vi "UHR-Fleezers Control (host) - Lorentz v4.vi"() -> ()   [LabVIEW 2014] (continued)
  out "Amp current":dbl[](graph)=[0.0169526657918025, 0.016960112308114644, 0.0169526657918025, 0.016960112308114644, 0.016932645649586246, 0.01696502578814028, 0.016922727134006547, 0.01697497482222945, 0.016955534531693243, 0.016920682393871657, 0.016913052766502658, 0.016956877346110188, 0.01690490432447257, 0.016908047730948596, 0.016886989959410157, 0.0168990142521437, 0.016891079439679938, 0.016886379589220638, 0.016868465224158226, 0.016933408612323148, 0.01688827173680815, 0.01690227973265763, 0.016862422559281977, 0.016931455427716683, 0.01689678640095195, 0.016911008026367767, 0.016896206549271906, 0.01695397808770997, 0.016912045655689947, 0.016928769798882796, 0.0169044770653399, 0.01693642994476127, 0.016903012176885054, 0.01690923795281816, 0.016908627582628635, 0.016958189642017656, 0.0169203772087769, 0.016929624317148124, 0.01689678640095195, 0.016945371868037736, 0.01693932920316149, 0.016923978392895066, 0.016900112918484835, 0.016959105197301934, 0.01693551438947699, 0.016914761803033314, 0.016874019592882858, 0.016916684469130302, 0.016878353221228447, 0.016893490401928547, 0.01686446729941687, 0.01691998046815371, 0.016895077364421293, 0.016919797357096856, 0.016901242103335445, 0.016928983428449125, 0.016912137211218377, 0.016924344615008777, 0.016907071138645362, 0.016948728904080095, 0.01691830195013253, 0.016923215430158164, 0.01688412121951941, 0.016954222235785774, 0.016917874690999864, 0.016929868465223933, 0.017037171544541534, 0.017055513168736606, 0.01704351939451254, 0.01703344828638546, 0.017046937467573853, 0.017029999694814675, 0.017005127109591737, 0.017014557329019818, 0.017042481765190357, 0.01701828058717589, 0.01702325510422048, 0.01703155613879795, 0.017028443250831398, 0.017003631702627413, 0.017003540147098987, 0.017018677327799075, 0.017034058656574983, 0.017009674367503662, 0.017002533036286276, 0.017015076143680908, 0.017031495101779, 0.017036103396709874, 0.017019562364573883, 0.01703680532242782, 0.01703247169408223, 0.017042023987548217, 0.017036347544785682, 0.017039704580828038, 0.017048371837519224, 0.017023987548447903, 0.017018555253761176, 0.01701858577227065, 0.05867714468825214, 0.05870891445661666, 0.058683095797599956, 0.05870555742057429, 0.058757133701588735, 0.058661000396739334, 0.05859691152683975, 0.05860075685903373, 0.058646565141757194, 0.05849485763115201, 0.05836561174352117, 0.05846021912289676, 0.05851405377361242, 0.058334055604723, 0.05814590899380348, 0.05832355723746325, 0.05841291543320897, 0.058184301278724274, 0.0581402935880599, 0.05840501113925468, 0.058464674825280255, 0.05835297708059811, 0.05824994659260716, 0.058513657032989226, 0.058697958311714774, 0.05858626056703263, 0.058617084261603385, 0.05881652272102902, 0.058878688924831626, 0.0588497268593389, 0.05885311441389074, 0.05887240211187957, 0.058940702536086846, 0.05897109897152494, 0.05889873958555736, 0.05887862788781267, 0.0589223303933823, 0.058909298989836045, 0.058916440321053434, 0.05885915707876699, 0.058968779564804764, 0.05885961485640912, 0.05876015503402685, 0.05881301309243928, 0.05886797692800556, 0.05875923947874257, 0.05869737846003473, 0.05872920926541819, 0.058807306131167275, 0.058688192388682454, 0.05864888454847737, 0.058773033845025725, 0.05883294167912711, 0.05877095858638136, 0.05871828363902579, 0.05878093813898001, 0.0589785149693276, 0.058929837946713394, 0.05889736625263094, 0.058995330668048886, 0.059074068422496955, 0.05902313303018152, 0.05905365153965752, 0.05902941984313356, 0.05876702169865896, 0.05880504776146604, 0.058806085390788236, 0.05879586169011377, 0.05884539323099332, 0.0588626972258662, 0.05887383648182495, 0.05881914731284396, 0.058912625507368935, 0.05881188390758866, 0.05869289223914176, 0.05873934141056422, 0.05880053102206359, 0.058644154179508586, 0.05851768547624006, 0.058613818781089455, 0.058685048982206424, 0.058522659993284654, 0.05842268135624129, 0.05860997344889547, 0.05869811090426215, 0.058628986480299024, 0.05857280190435372, 0.05869985045930229, 0.058889126255072415, 0.05879457991271578, 0.058788689840386904, 0.05892318491164763, 0.058971831415752365, 0.05892013306070003, 0.05893545335245698, 0.058890041810356696, 0.05878170110171691, 0.058839197973569686, 0.05883425397503458, 0.05883999145481606, 0.058881496627703415, 0.058851222266303224, 0.058815057832574166, 0.058749748222295534, 0.05883022553178374, 0.05875231177709152, 0.058630390331734915, 0.05871446882534128, 0.0587492904446534, 0.05856462294381415, 0.05845246742148986, 0.05858781701101591, 0.058693929868463945, 0.05851161229285434, 0.05842631305886894, 0.058632129886775054, 0.05872634052552745, 0.05861891537217195, 0.058535142063660325, 0.058678090762045894, 0.058843440046386856, 0.05878841517380163, 0.05875688955351293, 0.058908078249457006, 0.05898879970702102, 0.058959288308357734, 0.058988036744284114, 0.05898190252387944, 0.058596240119631285, 0.058748527481916495, 0.05874556718649733, 0.058761345255896415, 0.05880101931821521, 0.0588375194555485, 0.058903530991545085, 0.0587775200659187, 0.058887234107484906, 0.058839869380778155, 0.058704184087647875, 0.058698568681904296, 0.058713827936642295, 0.0585772576067372, 0.05845738090151549, 0.05850675984984766, 0.05861015655995234, 0.058485671559799744, 0.05842185735648543, 0.058601214636675864, 0.058648121585740474, 0.05859996337778734, 0.05855214087343846, 0.058672566911830745, 0.05884759056367559, 0.05878975798821857, 0.05877803888057979, 0.05885317545090969, 0.058908474990080194, 0.05888726462599438, 0.05890273751029871, 0.058803399761954346, 0.05871681875057094, 0.05878859828485848, 0.058835230567337804, 0.05886474196600109, 0.0589122898037647, 0.05887401959288179, 0.058873134556106994, 0.05876183355204803, 0.05887066255683944, 0.05875139622180725, 0.0586343577379668, 0.05867735831781847, 0.05873665578173034, 0.0585823541978197, 0.058473769341104105, 0.0585251319925522, 0.058599078341012543, 0.05843836787011195, 0.058349772637103135, 0.05851222266304386, 0.058603686635943425, 0.05852912991729356, 0.05853346354563915, 0.0586587725455476, 0.05880602435376927, 0.05876897488326542, 0.05873751029999567, 0.05881136509292758, 0.05890054017761644, 0.058819757683033484, 0.05879860835596661, 0.05880217902157531, 0.05889974669637006, 0.05896551408429084, 0.058984923856317574, 0.05896411023285493, 0.05903811761833423, 0.059025818659015405, 0.05908288827173551, 0.05897918637653608, 0.059064699240087816, 0.05897958311715927, 0.05885155796990746, 0.05884398937955741, 0.05889040803247041, 0.05873070467238251, 0.05861577196569592, 0.058758232367929875, 0.05888384655293307, 0.05866118350779621, 0.05851628162480418, 0.05870332956938255, 0.05880050050355412, 0.058731589709157324, 0.05870787682729447, 0.058827570421459335, 0.058956511123995414, 0.058872737815483814, 0.058847376934109255, 0.058931089205601916, 0.05896514786217713, 0.058957976012450265, 0.05900302133243683, 0.05900717184972557, 0.06101351969969651, 0.06100839259010454, 0.0610315866573063, 0.06104242072817028, 0.061070741904964004, 0.061021759697255026, 0.06087478255561864, 0.06096603289895187, 0.061050904873804594, 0.06088381603442353, 0.060784295175022304, 0.06089385662404114, 0.06096615497298976, 0.0607882320627447, 0.0605131076998186, 0.06074556718649726, 0.06088857692190178, 0.06070140690328549, 0.0607113254188652, 0.060980132450329766, 0.06108334604937759, 0.06106183050019703, 0.0610269173253565, 0.06115659047211998, 0.06127973265785563, 0.061202185125277114, 0.06119818720053577, 0.06126438184758922, 0.06133845027008745, 0.0613045747245691, 0.06130579546494813, 0.06127933591723245, 0.05855381939145965, 0.05864778588213623, 0.05864717551194672, 0.05865880306405707, 0.05868761253700241, 0.058670949430828526, 0.05869023712881735, 0.05858568071535258, 0.05865987121188873, 0.058558824427013705, 0.05844840845972956, 0.05845713675343968, 0.05853523361918876, 0.0584093142490908, 0.05830329294717119, 0.05836045411541973, 0.05842518387401832, 0.05830616168706193, 0.058225074007384206, 0.05840299691762928, 0.05847492904446419, 0.058402478102968176, 0.058411206396678315, 0.05852949613940728, 0.058743308816796104, 0.058691610461743766, 0.05866734824671034, 0.05872603534043269, 0.05876793725394323, 0.05870751060518076, 0.05876030762657424, 0.05872774437696335, 0.058540604876856535, 0.05860780663472268, 0.05859538560136596, 0.05858815271462014, 0.05863768425549967, 0.0585609912411865, 0.05847074800866599, 0.058447645496992655, 0.05850093081453774, 0.05836039307840078, 0.05823578600421028, 0.058302194280830055, 0.05836890774254458, 0.05820865504928613, 0.05803341776787497, 0.05822223578600294, 0.058326456495863474, 0.05810513626514355, 0.05803088473158845, 0.058302224799339525, 0.05838605914487009, 0.05830237739188691, 0.05823041474654251, 0.05844843897823903, 0.058613361003447315, 0.05853691213720995, 0.05851008636738054, 0.05862434766685867, 0.05869426557206819, 0.05865959654530345, 0.058693014313179664, 0.05867390972624769, 0.058459608752707254, 0.058497940000609094, 0.058514297921688226, 0.05845851008636611, 0.058465498825036114, 0.05839936521500163, 0.05831144138920129, 0.05836378063295261, 0.058509659108247875, 0.05833979308450448, 0.05816058839686143, 0.05820911282692826, 0.058273018585771004, 0.058127506332589465, 0.05791500595110811, 0.058098239082001964, 0.05819550157170197, 0.05795974608599991, 0.05790282906582718, 0.05815613269447793, 0.05821353801080229, 0.05813074129459392, 0.05802249214148255, 0.0582559892574834, 0.05843949705496257, 0.058309305093537954, 0.05832450331125701, 0.0584761803033527, 0.058528916287727224, 0.058529068880274614, 0.05852293465986993, 0.058511825922420664, 0.05836075930051449, 0.05838044373912651, 0.05834656819360815, 0.0583083590197442, 0.05836790063173187, 0.0583271889400909, 0.05821387371440652, 0.05820007934812337, 0.05828766747031948, 0.05810458693197297, 0.05798095645008572, 0.058052858058411164, 0.058106570635088915, 0.057952635273292, 0.05776818140201908, 0.05797247230445139, 0.058080294198430076, 0.057839930417797156, 0.057788201544235335, 0.058037812433239494, 0.058113742484815774, 0.05804470961638108, 0.05790942106387399, 0.05814114810632523, 0.05830320139164276, 0.05820310068056149, 0.05820941801202303, 0.05836936552018671, 0.05845033112582654, 0.0584423657948533, 0.05845237586596143, 0.05843824579607405, 0.06618018127994545, 0.06624231696523857, 0.06621686452833558, 0.066234138004699, 0.06623569444868228, 0.0661422162541573, 0.06606472975859774, 0.0660725424970236, 0.06616202276680722, 0.06602536088137372, 0.06589510788293017, 0.06595434430982307, 0.0660394909512611, 0.06588830225531703, 0.06573943296609311, 0.0658894619586771, 0.06600634784997017, 0.06578795739615995, 0.0657112338633373, 0.06595065157017647, 0.06601303140354542, 0.0659321878719435, 0.06585607470931037, 0.06604416028321092, 0.06619989623706693, 0.06608703878902471, 0.06609637745292435, 0.06622721030304794, 0.06632587664418385, 0.06631598864711362, 0.06632871486556512, 0.06636286507766875, 0.05736872463148777, 0.0574271675771343, 0.05746177556688008, 0.05744721823786003, 0.057509079256567876, 0.05756801049836602, 0.05761238441114413, 0.057530045472577875, 0.05764592425305824, 0.057585131382182055, 0.05749800103762809, 0.05745878475295143, 0.05749580370494582, 0.0574180120242915, 0.05724723044526382, 0.057307199316384165, 0.05737723929563157, 0.05723194067201635, 0.05720749534592608, 0.05727069917905087, 0.057326944792015125, 0.05728937650685018, 0.05714386425366863, 0.05728485976744773, 0.05739963988158695, 0.05727668080690817, 0.057335856196782116, 0.057406933805351716, 0.05750538651692127, 0.05751487777336831, 0.05750791955320778, 0.05751237525559128, 0.0579019135105429, 0.057950621051666575, 0.05796240119632431, 0.05800354014709795, 0.05807751701406777, 0.05802401806695634, 0.05797326578569777, 0.05794228949857964, 0.05806445509201205, 0.057933103427227364, 0.05782091738639359, 0.05785024567400003, 0.05789986877040799, 0.05782879116183841, 0.05771279030732014, 0.057787591174045805, 0.05788631855220066, 0.05776650288399789, 0.05774541459394999, 0.05785424359874138, 0.05789892269661424, 0.057857509079255326, 0.05777422406689533, 0.05784292123172579, 0.05801474044007564, 0.057907681508833846, 0.05787569811090301, 0.057927182836389014, 0.05803646961882255, 0.05800271614734211, 0.05796234015930536, 0.0580202642902908, 0.05792464980010252, 0.05796942045350379, 0.05797836237678025, 0.05799984740745135, 0.0580758384960466, 0.058039918210393344, 0.05797555467390846, 0.057967711416973135, 0.05806714072084593, 0.05790752891628647, 0.05781246375926873, 0.05789739677114044, 0.05790667439802114, 0.05778249458296332, 0.05767168187505598, 0.05778655354472362, 0.05789397869807913, 0.0577122104556401, 0.05768956572160892, 0.05784655293435343, 0.05788677632984279, 0.05784020508438243, 0.05778206732383066, 0.057885952330086934, 0.05803570665608565, 0.05795416119876579, 0.057946226386302035, 0.05803753776665421, 0.05812762840662736, 0.058096713156528174, 0.05809207434308782, 0.058102298043762275, 0.05806143375957393, 0.05811123996703875, 0.05805520798364082, 0.058111789300209306, 0.05817474898525829, 0.0580753196813855, 0.058212408825951675, 0.058142857142855886, 0.058066560869165895, 0.05824359874263614, 0.05785604419080046, 0.05796322519608016, 0.05793871883297095, 0.05772667622913172, 0.05788586077455851, 0.05762819299905268, 0.05773351237525435, 0.05785674611651842, 0.057791344950711344, 0.05774202703939816, 0.057862514114809395, 0.05796548356578139, 0.058087252418590606, 0.05802334665974788, 0.058187139500105546, 0.05831589709158477, 0.058206366161075426, 0.05834241767631942, 0.058355296487318284, 0.05832770775475199, 0.058404431287574644, 0.05832322153385901, 0.057956236457410173, 0.05807815790276677, 0.05797738578447702, 0.05809973448896629, 0.058119327372049896, 0.05800067140720722, 0.058170628986479025, 0.05800714133121612, 0.058036286507765704, 0.05824527726065733, 0.057814294869837295, 0.05800772118289617, 0.057920133060700076, 0.057680990020446146, 0.0579498275704202, 0.05751332132938503, 0.05765117343668811, 0.05784679708242925, 0.05769692068239263, 0.057814172795799416, 0.05789358195745595, 0.05794454786828085, 0.05816174810022152, 0.058005859553818144, 0.05820203253272983, 0.05834952848902733, 0.05815979491561506, 0.058378124332406335, 0.05834629352702286, 0.058285500656146676, 0.058417096469007175, 0.05825724051637192, 0.00451747184667494, 0.0045178380687886524, 0.004530625324259094, 0.004513870662556772, 0.004487319559312655, 0.00448576311532938, 0.004487960448011651, 0.004507248146000482, 0.004523758659626995, 0.004526871547593547, 0.004501358073671614, 0.00451976073488564, 0.004508896145512186, 0.004513260292367252, 0.004468642231513346, 0.004494369335001612, 0.0045054170354319216, 0.004491683706167724, 0.004517441328165464, 0.004521317178868915, 0.0044969328897975945, 0.00449894711142301, 0.004529099398785295, 0.004523361919003807, 0.0044921414838098635, 0.004499893185216767, 0.004504501480147641, 0.004517807550279176, 0.004495254371776414, 0.0045184179204686955, 0.004501815851313753, 0.004515915402691664, 0.00451518295846424, 0.004509201330606945, 0.004514664143803148, 0.0045286111026336786, 0.0045125583666493045, 0.004529648731955862, 0.0045194860683003555, 0.004531632435071802, 0.004528153324991538, 0.0045108493301186485, 0.004501663258766373, 0.004521774956511055, 0.004506179998168821, 0.004507034516434149, 0.00453736991485329, 0.004532212286751846, 0.004493789483321567, 0.004512192144535593, 0.004510544145023889, 0.0045054170354319216, 0.004482680745872304, 0.004494644001586895, 0.004525864436780839, 0.004527573473311494, 0.004488357188634839, 0.004510727256080744, 0.004482375560777544, 0.004494460890530039, 0.004530747398296998, 0.004528153324991538, 0.0045117038483839765, 0.004530106509598003, 0.004536667989135342, 0.004536973174230101, 0.004502456740012749, 0.004504898220770829, 0.0045134128849146325, 0.004523422956022759, 0.004539872432630321, 0.004540787987914601, 0.004515091402935813, 0.0045239112521743745, 0.0045441755424664365, 0.00454490798669386, 0.004507156590472053, 0.0045294045838800544, 0.00454506057924124, 0.0045275429548020186, 0.004537614062929097, 0.004557512131107447, 0.00454261909848316, 0.004543076876125301, 0.004543870357371677, 0.004556077761162075, 0.004526810510574595, 0.0045342570268867375, 0.004537766655476477, 0.004520157475508827, 0.004520004882961447, 0.004536881618701674, 0.004530930509353854, 0.0045216223639636755, 0.004538926358836565, 0.004546220282601328, 0.00453050325022119, 0.004536637470625865, 0.004538438062684949, 0.004536362804040581, 0.004521897030548959, 0.00454261909848316, 0.004539201025421849, 0.004540604876857745, 0.004533066805017174, 0.0045422528763694485, 0.0045353251747183975, 0.004539353617969229, 0.004543412579729536, 0.00453172399060023, 0.004509842219305941, 0.004526566362498786, 0.004526139103366122, 0.004507553331095241, 0.004505935850093013, 0.004508407849360569, 0.004485183263649335, 0.004518478957487648, 0.004524857325968131, 0.004523148289437475, 0.0044967192602312625, 0.004523636585589091, 0.004524063844721755, 0.004527634510330446, 0.004510238959929129, 0.4378774681844542, 1.1794734031189942, 1.1789416180913743, 1.1792670369579177, 1.179584032715845, 1.1793981749931346, 1.1797783135471682, 1.1800726035340454, 1.1801462141789023, 1.1801267433698555, 1.1802436597796602, 1.1802706991790544, 1.1801345561082817, 1.1798594622638647, 1.1805548570207856, 1.1800792870876216, 1.180210882900482, 1.1803491927854268, 1.180768028809476, 1.1809785149693315, 1.180827448347424, 1.1799802240058617, 1.179896664326917, 1.180044587542347, 1.1803296304208517, 1.1806996978667577, 1.1806953337199022, 1.1803043610950055, 1.1801087679677742, 0.004506088442640393, 0.0045059968871119654, 0.004491286965544535, 0.004513748588518868, 0.004526596881008263, 0.004524460585344943, 0.004505478072450874, 0.004522293771172147, 0.004515152439954764, 0.004519241920224548, 0.004482039857173309, 0.0044971465193639265, 0.004498001037629254, 0.0045084994048889965, 0.004515121921445288, 0.004521164586321535, 0.004507797479171049, 0.004512009033478736, 0.004528153324991538, 0.00452836695455787, 0.004506271553697249, 0.004514511551255768, 0.004501449629200041, 0.004526291695913503, 0.004532151249732895, 0.0045214087343973435, 0.004510788293099696, 0.004531937620166562, 0.004528855250709486, 0.004528794213690534, 0.004525589770195555, 0.0045243385113070385, 0.0045346842860194015, 0.004532090212713943, 0.004516800439466468, 0.004500595110934714, 0.004492385631885671, 0.004502883999145414, 0.004513321329386205, 0.004511154515213408, 0.004502151554917989, 0.00450840784936057, 0.004521225623340487, 0.004522293771172147, 0.004514236884670484, 0.004512466811120877, 0.004515396588030573, 0.004535660878322634, 0.004548966948454168, 0.004552293465987052, 0.004536149174474249, 0.004540818506424077, 0.00451960814233826, 0.004544022949919057, 0.004505386516922445, 0.004527726065858875, 0.004533524582659314, 0.0045262611774040265, 0.004496505630664931, 0.00451686147648542, 0.004499343852046198, 0.00450672933133939, 0.004491500595110867, 0.004498580889309298, 0.004497970519119779, 0.004507980590227906, 0.004519058809167692, 0.00452714621417883, 0.004487655262916892, 0.004493240150150999, 0.004516464735862233, 0.0045340433973204055, 0.004503250221259125, 0.004529648731955862, 0.00453141880550547, 0.004522385326700575, 0.004505172887356113, 0.0045101474044007, 0.004472151860103085, 0.004482497634815448, 0.004503311258278077, 0.004508224738303713, 0.004481734672078548, 0.004476821192052912, 0.00448133793145536, 0.0044705343791008574, 0.004461653492843343, 0.004484511856440865, 0.0044708090456861424, 0.004477065340128721, 0.004498916592913535, 0.0045179906613360315, 0.004504165776543405, 0.004503036591692794, 0.004511093478194457, 0.004509109775078518, 0.004491317484054011, 0.0044997100741599105, 0.004502395702993798, 0.004528489028595774, 0.004513290810876728, 0.004509414960173277, 0.004487166966765276, 0.004490585039826587, 0.004505539109469825, 0.004507461775566813, 0.004499343852046199, 0.00451350444044306, 0.004525437177648175, 0.004515549180577952, 0.004484939115573528, 0.004506698812829914, 0.004477126377147673, 0.004498092593157682, 0.0045196996978666875, 0.004511307107760788, 0.004494491409039515, 0.004516220587786424, 0.00448377941221344, 0.0044651020844141305, 0.004472701193273654, 0.004486190374462044, 0.004484633930478769, 0.0044800866725668445, 0.004447065645313817, 0.004473952452162169, 0.004472640156254701, 0.004481032746360601, 0.004478347117526713, 0.004480666524246888, 0.004484664448988244, 0.004488845484786455, 0.004467726676229066, 0.004478499710074093, 0.004464552751243563, 0.004477187414166625, 0.004497085482344975, 0.0044811548203985046, 0.0044492629779960885, 0.00446327097384557, 0.0044792321543015165, 0.004483260597552348, 0.004469466231269198, 0.004472518082216797, 0.004504104739524454, 0.00449125644703506, 0.00450169377727585, 0.004497054963835498, 0.00446632282479317, 0.00447212134159361, 0.004497482222968162, 0.004509384441663801, 0.004476973784600293, 0.004497634815515542] caption="Most Recent Time Trace"
  out "Values":dbl[](array[numeric])=[nan, nan, 0.010932615131076998, nan, nan, 0.010855525376140629, -inf, 0.0332469252601703, -inf, 0.03308018738364819, nan, nan, 0.005625431073946348, 0.01681456484606091, 0.0867058284381119, 1.1533333333333333]
  out "All Signals":waveform(dbl)[](graph)=[{"t0"=timestamp(317.7000000000063 s since 1904-01-01), "dt"=0.15, "Y"=[0.0, 0.0], "attributes"=variant("NI_ChannelName"=variant(string "APD 1"))}, {"t0"=timestamp(317.7000000000063 s since 1904-01-01), "dt"=0.15, "Y"=[0.0, 0.0], "attributes"=variant("NI_ChannelName"=variant(string "APD 2"))}, {"t0"=timestamp(317.7000000000063 s since 1904-01-01), "dt"=0.15, "Y"=[0.0, 0.0], "attributes"=variant("NI_ChannelName"=variant(string "APD 3"))}, {"t0"=timestamp(317.7000000000063 s since 1904-01-01), "dt"=0.15, "Y"=[nan, nan], "attributes"=variant("NI_ChannelName"=variant(string "T1 Y"))}, {"t0"=timestamp(317.7000000000063 s since 1904-01-01), "dt"=0.15, "Y"=[nan, nan], "attributes"=variant("NI_ChannelName"=variant(string "T1 X"))}, {"t0"=timestamp(317.7000000000063 s since 1904-01-01), "dt"=0.15, "Y"=[0.010935636463514926, 0.01092959379863868], "attributes"=variant("NI_ChannelName"=variant(string "T1 Sum"))}, {"t0"=timestamp(317.7000000000063 s since 1904-01-01), "dt"=0.15, "Y"=[nan, nan], "attributes"=variant("NI_ChannelName"=variant(string "T2 Y"))}, {"t0"=timestamp(317.7000000000063 s since 1904-01-01), "dt"=0.15, "Y"=[nan, nan], "attributes"=variant("NI_ChannelName"=variant(string "T2 X"))}, {"t0"=timestamp(317.7000000000063 s since 1904-01-01), "dt"=0.15, "Y"=[0.010837214270454837, 0.010873836481826035], "attributes"=variant("NI_ChannelName"=variant(string "T2 Sum"))}, {"t0"=timestamp(317.7000000000063 s since 1904-01-01), "dt"=0.15, "Y"=[-inf, -inf], "attributes"=variant("NI_ChannelName"=variant(string "T1 FB X"))}, {"t0"=timestamp(317.7000000000063 s since 1904-01-01), "dt"=0.15, "Y"=[0.03323676259651433, 0.033257087923825326], "attributes"=variant("NI_ChannelName"=variant(string "T1 FB Sum"))}, {"t0"=timestamp(317.7000000000063 s since 1904-01-01), "dt"=0.15, "Y"=[-inf, -inf], "attributes"=variant("NI_ChannelName"=variant(string "T2 FB X"))}, {"t0"=timestamp(317.7000000000063 s since 1904-01-01), "dt"=0.15, "Y"=[0.033094546342356174, 0.03306582842493926], "attributes"=variant("NI_ChannelName"=variant(string "T2 FB Sum"))}, {"t0"=timestamp(317.7000000000063 s since 1904-01-01), "dt"=0.15, "Y"=[nan, nan], "attributes"=variant("NI_ChannelName"=variant(string "T3 Y"))}, {"t0"=timestamp(317.7000000000063 s since 1904-01-01), "dt"=0.15, "Y"=[nan, nan], "attributes"=variant("NI_ChannelName"=variant(string "T3 X"))}, {"t0"=timestamp(317.7000000000063 s since 1904-01-01), "dt"=0.15, "Y"=[0.005610065004425081, 0.005640797143467409], "attributes"=variant("NI_ChannelName"=variant(string "T3 Sum"))}, {"t0"=timestamp(317.7000000000063 s since 1904-01-01), "dt"=0.02, "Y"=[0.015748031496062992, 0.015748031496062992, 0.015748031496062992, 0.015748031496062992, 0.015748031496062992, 0.015748031496062992, 0.015748031496062992, 0.015748031496062992, 0.015873015873015872, 0.023622047244094488, 0.015873015873015872, 0.015748031496062992, 0.023622047244094488, 0.015748031496062992, 0.015748031496062992], "attributes"=variant("NI_ChannelName"=variant(string "PSD X"))}, {"t0"=timestamp(317.7000000000063 s since 1904-01-01), "dt"=0.02, "Y"=[0.08661417322834646, 0.08661417322834646, 0.08661417322834646, 0.08661417322834646, 0.08661417322834646, 0.08661417322834646, 0.08661417322834646, 0.08661417322834646, 0.0873015873015873, 0.08661417322834646, 0.0873015873015873, 0.08661417322834646, 0.08661417322834646, 0.08661417322834646, 0.08661417322834646], "attributes"=variant("NI_ChannelName"=variant(string "PSD Y"))}, {"t0"=timestamp(317.7000000000063 s since 1904-01-01), "dt"=0.02, "Y"=[1.1545454545454545, 1.1545454545454545, 1.1545454545454545, 1.1545454545454545, 1.1545454545454545, 1.1545454545454545, 1.1545454545454545, 1.1545454545454545, 1.1454545454545455, 1.1545454545454545, 1.1454545454545455, 1.1545454545454545, 1.1545454545454545, 1.1545454545454545, 1.1545454545454545], "attributes"=variant("NI_ChannelName"=variant(string "PSD Sum"))}]
  in  "PSD downsample":dbl=1.0 caption="PSD Downsample" min=1.0 max=5.0
  in  "Signals to Plot":i32(listbox)=18
  out "Trap Disp. Freq. (Hz)":dbl=6.666666666666667 caption="Freq. (Hz)" format="%#_6p"
  out "Display Period (s)":dbl=0.15 caption="Period (s)" format="%#_6p"
  in  "Trap Disp. Downsample":dbl=10000.0 caption="Downsample" max=20000.0
  in  "APD Disp. Scale":dbl=0.1 caption="Scale (Divide,\nfor above plot only)"
  in  "APD Disp. Downsample":dbl=150.0 caption="Integrate" max=300.0
  out "APD Display Freq. (Hz)":dbl=6.666666666666667 caption="Freq. (Hz)"
  out "APD Display Period (s)":dbl=0.15 caption="Period (s)"
  out "FFT 1":cluster{"f0":dbl, "df":dbl, "magnitude":dbl[]}[](graph)=[{"f0"=0.0, "df"=3.3333333333333335, "magnitude"=array[10000 elements]}, {"f0"=0.0, "df"=3.3333333333333335, "magnitude"=array[10000 elements]}]
  out "FFT 2":cluster{"f0":dbl, "df":dbl, "magnitude":dbl[]}[](graph)
  in  "FFT 1 Choice 1":u16(ring) items=["T1 Y", "T1 X", "T1 Sum", "T2 Y", "T2 X", "T2 Sum", "T1 FB X", "T1 FB Sum", "T2 FB X", "T2 FB Sum", "PSD Y", "PSD X", "PSD Y Sum", "none"]
  in  "FFT 2 Choice 1":u16(ring)=13 items=["T1 Y", "T1 X", "T1 Sum", "T2 Y", "T2 X", "T2 Sum", "T1 FB X", "T1 FB Sum", "T2 FB X", "T2 FB Sum", "PSD Y", "PSD X", "PSD Y Sum", "none"]
  in  "FFT 1 Choice 2":u16(ring)=1 items=["T1 Y", "T1 X", "T1 Sum", "T2 Y", "T2 X", "T2 Sum", "T1 FB X", "T1 FB Sum", "T2 FB X", "T2 FB Sum", "PSD Y", "PSD X", "PSD Y Sum", "none"]
  in  "FFT 2 Choice 2":u16(ring)=13 items=["T1 Y", "T1 X", "T1 Sum", "T2 Y", "T2 X", "T2 Sum", "T1 FB X", "T1 FB Sum", "T2 FB X", "T2 FB Sum", "PSD Y", "PSD X", "PSD Y Sum", "none"]
  in  "Compute FFT":bool
  in  "Reset FFT":bool
  in  "# Spectra to Ave.":dbl=25.0
  out "Ave. Time (s)":dbl=7.5
  out "1 Channel":waveform(dbl)(graph)={"t0"=timestamp(0 s since 1904-01-01), "dt"=1.4999999999999999e-05, "Y"=array[20000 elements], "attributes"=variant("NI_ChannelName"=variant(string "T1 X"))}
  out "Slow mean":dbl=nan format="%0.2f"
  in  "Slow mean N ave.":dbl=1.0 min=1.0 step=1.0
  out "Mean Intensity":dbl=nan
  out "Sigma":dbl=nan
  out "Sigma/Mean":dbl=nan
  in  "Subtract mean":bool
  in  "High Res. Display":u16(ring)=1 items=["T1 Y", "T1 X", "T1 Sum", "T2 Y", "T2 X", "T2 Sum", "T1 FB X", "T1 FB Sum", "T2 FB X", "T2 FB Sum", "PSD Y", "PSD X", "PSD Y Sum"]
  in  "Tab Control":T7(tab)=enum."Trap Control (RF)"
  in  "Visa resource for valves":refnum<visa-resource-name>="COM10"
  in  "Cursor control":cluster{"X":bool, "Y":bool}
  in  "Trap 3 (ON/OFF)":bool=TRUE
  in  "Maximum Delta\n(MHz)":dbl=30.0
  in  "T3 Y (V)":dbl min=0.0 max=10.0 step=1.0 format="%#_6f"
  in  "T3 X (V)":dbl=3.0 min=0.0 max=10.0 step=1.0 format="%#_6f"
  in  "Shunt 1":bool caption="Inject Pump 3"
  in  "manual raster set":u16(ring) items=["offset", "user-defined", "basepaire step", "user-defined 2", "user-defined 3", "user-defined 4"]
  in  "move Con X?":bool
  in  "Symmetric?":bool
  out "Laser Intensity Low (bugs to fix)":bool
  out "Good freq?":bool=TRUE
  in  "T2 calibration":T8 {"T2 kappa_x (pN/nm)" min=0.0 step=0.001 format="%#_2g"; "T2 offset_x (mV)" format="%#_2g"; "T2 alpha_x (nm/V)" step=10.0 format="%#_3g"}
  in  "T1 calibration":T9 {"T1 kappa_x (pN/nm)" min=0.0 step=0.001 format="%#_2g"; "T1 offset_x (mV)" format="%#_2g"; "T1 alpha_x (nm/V)" step=10.0 format="%#_3g"}
  in  "Blue FB Setpoint (mV)":dbl=90.0
  in  "Blue Laser ON":bool
  in  "11":bool
  out "Stage Moving":bool
  in  "Read Cal":bool
  in  "Speed (nm/s)":dbl=100.0
  in  "Furthest Withdraw (MHz)":dbl=15.0
  in  "Round T1 X":bool caption="Round"
  in  "Cal sets to save":u32=25 min=1 step=1
  in  "Trap 2 (ON/OFF)":bool=TRUE
  in  "Trap 1 (ON/OFF)":bool=TRUE
  in  "Save Calibration":bool
  out "Manipulating Trap":bool
  out "Buffer Status":dbl(slide) scale=0.0..1.0
  out "Overflow (data lost)":bool
  in  "Reset":bool
  out "Data Rate (Hz)":dbl=66666.66666666667 caption="Trap Data Rate (Hz)" format="%#_3p"
  out "Data Period (s)":dbl=1.4999999999999999e-05 caption="Trap Data Period (s)" format="%#_6p"
  in  "BD 1 Frequency 1 (MHz)":dbl=75.0 caption="T1 X (MHz)" min=60.0 max=90.0 step=1.0 format="%#_6p"
  in  "BD 1 Frequency 2 (MHz)":dbl=90.0 caption="T2 X (MHz)" min=60.0 max=90.0 step=1.0 format="%#_6p"
  in  "Round T2 X":bool caption="Round"
  in  "Trap Raster Scan":bool
  out "Raster Scanning...":bool
  in  "Trap Delta (MHz)":dbl=15.0
  in  "Setpoints (V)":cluster{"Set 1":dbl, "Set 2":dbl}={"Set 1"=0.9, "Set 2"=0.9}
  in  "Fish for Tether":bool
  in  "Red FB Setpoint (mV)":dbl=100.0
  in  "Confocal Linescan":bool
  in  "Confocal Image":bool
  in  "Green Laser ON":bool
  in  "AO1":dbl(slide)=5.709081392864773 caption="Confocal Y (V)" min=0.0 max=10.0 step=0.01 scale=0.0..10.0 scale format="%_1f"
  in  "AO2":dbl(slide)=4.827825251014741 caption="Confocal X (V)" min=0.0 max=10.0 step=0.01 scale=0.0..10.0 scale format="%_1f"
  in  "Green FB Setpoint (mV)":dbl=200.0
  in  "Red Laser ON":bool
  in  "Active Cal":bool
  out "A cal freq (Hz)":dbl=333.3333333333333 caption="Freq. (Hz)"
  in  "Laser interlacing mode":enum32{"Laser ON", "Laser OFF", "Interlace"}(radio)=enum."Interlace" caption="Laser interlacing mode (all lasers)"
  in  "Green Intensity % (FB OFF)":dbl=7.0 min=0.0 max=100.0 step=1.0
  in  "Shunt 2":bool caption="Inject Pump 3"
  out "Piezo trap cursor control":cluster{"X":dbl, "Y":dbl}[](graph)
  in  "Position Label 6":string="upper flow spot (5-hole)" caption="6"
  in  "Move to Position 6":bool
  in  "Set Position 6":bool
  in  "Position Label 5":string="central flow spot (UvrD)" caption="5"
  in  "Move to Position":bool
  in  "Position":dbl=1.0 min=1.0 max=10.0 step=1.0
  in  "Set Position":bool
  in  "Saved Stage Positions":dbl[][](array[numeric])=[[1.0, 0.0, 0.0, 0.0], [2.0, 0.47143, -1.65361, -0.02271], [3.0, 1.5, -0.5, 0.0], [4.0, -0.17227, -2.30048, -0.0394], [5.0, 1.5, -2.0, -0.02], [6.0, 0.0, 0.0, 0.0], [7.0, 0.0, 0.0, 0.0], [8.0, 0.0, 0.0, 0.0], [9.0, 0.0, 0.0, 0.0], [10.0, 0.0, 0.0, 0.0]]
  in  "Move to Position 5":bool
  in  "Position 1 Label":string="Lower capillary (DNA beads)" caption="1"
  in  "Set Position 1":bool
  in  "Set Position 2":bool
  in  "Set Position 3":bool
  in  "Set Position 4":bool
  in  "Move to Position 3":bool
  in  "Move to Position 4":bool
  in  "Move to Position 2":bool
  in  "Move to Position 1":bool
  in  "Position 2 Label":string="Upper capillary (ADig beads)" caption="2"
  in  "Position 3 Label":string="lower flow spot (ATP)" caption="3"
  in  "Position 4 Label":string="Dump beads" caption="4"
  in  "Set Position 5":bool
  out "Stage Control Serial Error":errorcluster
  in  "y nudge increment (um":dbl=0.5
  in  "-y":bool
  in  "+y":bool
  in  "x nudge increment (um)":dbl=0.5
  in  "-x":bool
  in  "+x":bool
  in  "-z":bool
  in  "+z":bool
  in  "z nudge increment (um)":dbl=0.5
  in  "Pressure Pump Voltage (+/-10V)":dbl
  in  "Use Harvard pumps\nfor beads (else Chemyx)":bool=TRUE
  in  "Tab Control 9":enum32{"Harvard Pumps", "Chemyx Pumps"}(tab)
  in  "Display On P3":bool caption="Display On"
  in  "Normal Flow Rate (ul/h) P3":dbl=800.0 caption="Normal Flow Rate (ul/h)"
  out "Flushing P3":bool caption="Flushing"
  in  "Retract Vol 1 (uL)":dbl=250.0 caption="Volume (uL)"
  in  "Retract Vol 3 (uL)":dbl=250.0 caption="Volume (uL)"
  in  "Retract Rate (uL/m)":dbl=2000.0
  in  "Retract Pump 1":bool
  in  "Retract Pump 3":bool
  in  "Stop Flow":bool
  in  "Start Flow":bool
  in  "Flush Sample":bool
  in  "Volume (uL)":dbl=100.0
  in  "Flush rate (uL/m)":dbl=100.0
  in  "Flow rate (uL/h)":dbl=100.0
  in  "Clear Volume":bool caption="Clear Infused Volume"
  in  "Flush Pump 3":bool
  in  "Volume (uL) P3":dbl=150.0 caption="Volume (uL)"
  in  "Flush rate (uL/m) P3":dbl=100.0 caption="Rate (uL/m)"
  out "Flushing P1":bool caption="Flushing"
  in  "Volume (uL) P1":dbl=100.0 caption="Volume (uL)"
  in  "Flush rate (uL/m) P1":dbl=100.0 caption="Rate (uL/m)"
  in  "Normal Flow Rate (ul/h) P1":dbl=600.0 caption="Normal Flow Rate (ul/h)"
  in  "Flush Pump 1":bool
  in  "Clear Volume P3":bool caption="Clear Infused Volume"
  in  "Clear Volume P1":bool caption="Clear Infused Volume"
  in  "Display On P1":bool caption="Display On"
  in  "All Pump Parameters":T10={"Pump 1"={"Diameter (mm)"=4.61, "Units"=4.0, "Volume"=100.0, "Rate"=25.0}, "Pump 2"={"Diameter (mm)"=4.61, "Units"=3.0, "Volume"=0.0, "Rate"=0.0}, "Pump 3"={"Diameter (mm)"=4.61, "Units"=4.0, "Volume"=100.0, "Rate"=800.0}}
  in  "Total Volume\nFlushed (uL)":dbl
  in  "Inject Pump 2":bool caption="Inject Pump 2\n(Flush Center)"
  in  "Flush Center Ch Rate (ul/m)":dbl=100.0
  in  "Flush Center Ch Volume (uL)":dbl=15.0
  in  "Pump pause delay (ms)":u32
  in  "Pump write delay (ms)":dbl=300.0
  in  "Ch 3 Inject Rate (ul/h)":dbl=800.0
  in  "Ch 3 Inject Volume (uL)":dbl=100.0
  in  "Ch 1 Inject Volume (uL)":dbl=100.0
  in  "Ch 1 Inject Rate (ul/h)":dbl=25.0
  out "Pump 1 cont disp":string="Right: DNA beads "
  out "Pump 3 cont disp":string="Left: ADig beads"
  in  "Read Harvard":bool
  out "read buffer":string
  out "Serial Settings:Number of Bytes at Serial Port":u32
  in  "write buffer":string
  in  "Tab Control 2":T11(tab)=enum."Feedback on Trap Position"
  in  "Update all trap values":bool
  out "Total Counts (ticks)":u16=600
  in  "Trap ON/OFF X or Y Amp?":bool=TRUE
  in  "Oscillate Set 1":bool
  in  "Trap 1 ON":bool
  in  "Number Interlace Sets":u8=3 min=1 max=3
  in  "DIO count 3 (ticks)":u16=200
  in  "DIO count 2 (ticks)":u16=200
  in  "DIO count 1 (ticks)":u16=200
  in  "BD 2 Amplitude 3 (%)":dbl min=0.0 max=45.0 step=1.0
  in  "BD 2 Amplitude 2 (%)":dbl min=0.0 max=45.0 step=1.0
  in  "BD 2 Amplitude 1 (%)":dbl min=0.0 max=45.0 step=1.0
  in  "BD 1 Amplitude 3 (%)":dbl min=0.0 max=50.0 step=1.0
  in  "BD 1 Amplitude 2 (%)":dbl=30.0 min=0.0 max=50.0 step=1.0
  in  "BD 1 Amplitude 1 (%)":dbl=30.0 min=0.0 max=50.0 step=1.0
  in  "BD 2 Frequency 3 (MHz)":dbl=26.0 min=0.0 max=40.0 step=0.1 format="%#_6p"
  in  "BD 1 Frequency 3 (MHz)":dbl=70.0 min=60.0 max=90.0 step=1.0 format="%#_6p"
  in  "BD 2 Frequency 2 (MHz)":dbl=26.0 min=0.0 max=40.0 step=0.1 format="%#_6p"
  in  "BD 2 Frequency 1 (MHz)":dbl=26.0 min=0.0 max=40.0 step=0.1 format="%#_6p"
